vi "add_data_raw_line_exp.vi"(8 "error in (no error)":errorcluster, 10 "add Data":i32[][][](array[numeric]), 11 "Experiment.lvclass in":refnum<class "Experiment.lvclass">) -> (0 "error out":errorcluster, 3 "Experiment.lvclass out":refnum<class "Experiment.lvclass">)   [LabVIEW 2020, in "Experiment.lvclass"]
uses:
  Experiment.lvclass
  Experiment.lvclass/Experiment.ctl
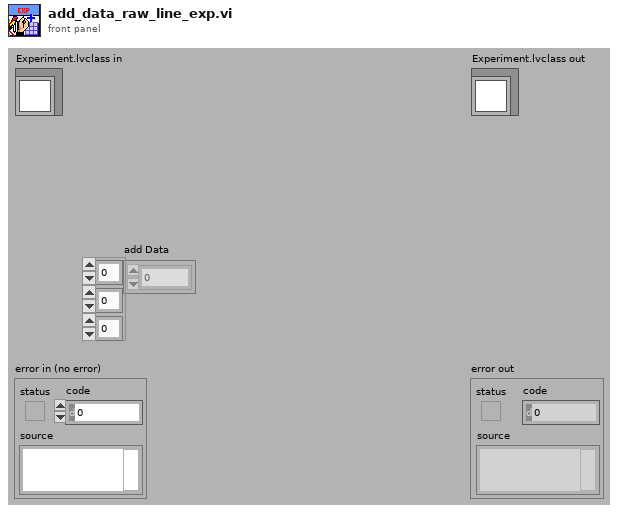
[diagram p1: front panel]
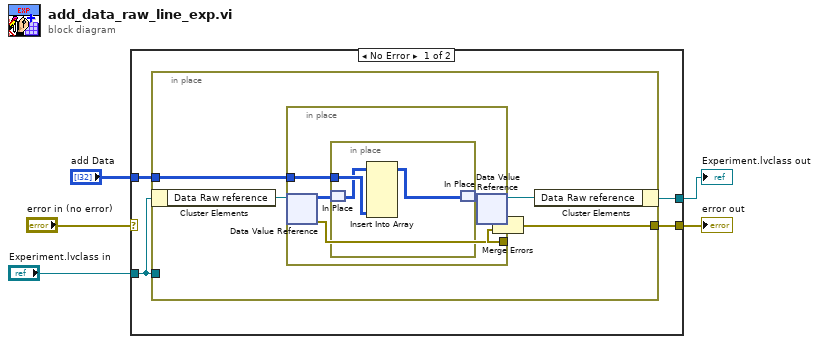
[diagram p0: block diagram]
diagram:
  n1 = case shown="No Error" "error in (no error)" {
    selector: "error in (no error)" -> [_ w23]
    tunnel: [w6 w23] -> w4
    tunnel: [w7 w24] -> w2
    tunnel: "Experiment.lvclass in" -> [w8 w24]
    tunnel: "add Data" -> [w9 _]
    frame No Error {
      n2 = in-place {
        in-place-border: w8 -> [_]
        in-place-border: w9 -> [w15]
        in-place-border: [w10] -> w6
        n3 = in-place-cluster #1(w8) -> ("Data Raw reference"=w14:refnum<data-value>)
        n4 = in-place {
          in-place-border: w15 -> [w19]
          in-place-border: [w16] -> w12
          n5 = in-place-dvr #2(w14) -> (w18:i32[][][][], w16:errorcluster)
          n6 = in-place {
            in-place-border: w19 -> [w22]
            n7 = in-place-match #3(w18) -> (w21:i32[][][][])
            n8 = Insert Into Array(array=w21, new element=w22) -> (w20:i32[][][][])  [unwired: 4 in]
            n9 = in-place-match #3(w20) -> (w17:i32[][][][])
          }
          n10 = in-place-dvr #2(w17) -> (w13:refnum<data-value>, w11:errorcluster)
        }
        n11 = Merge Errors(w11, w12) -> (w10:errorcluster)
        n12 = in-place-cluster #1("Data Raw reference"=w13) -> (w7:refnum<class "Experiment.lvclass">)
      }
    }
    frame Error {
    }
  }
  "error out" <- w4
  "Experiment.lvclass out" <- w2
